vi "Clear IP.vi"(8 "error in (no error)":errorcluster, 11 "Engine Simulation IP in":refnum<class "Engine Simulation IP.lvclass">) -> (0 "error out":errorcluster)   [LabVIEW 2013, in "Engine Simulation IP.lvclass"]
uses:
  Engine Simulation IP.lvclass
  Engine Simulation IP.lvclass/Engine Simulation IP.ctl
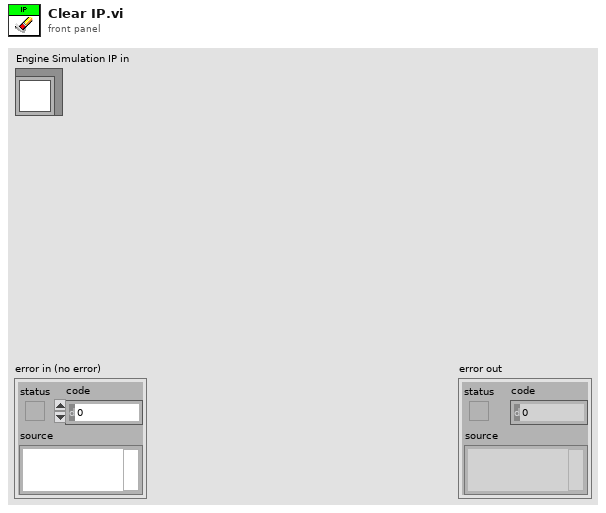
[diagram p1: front panel]
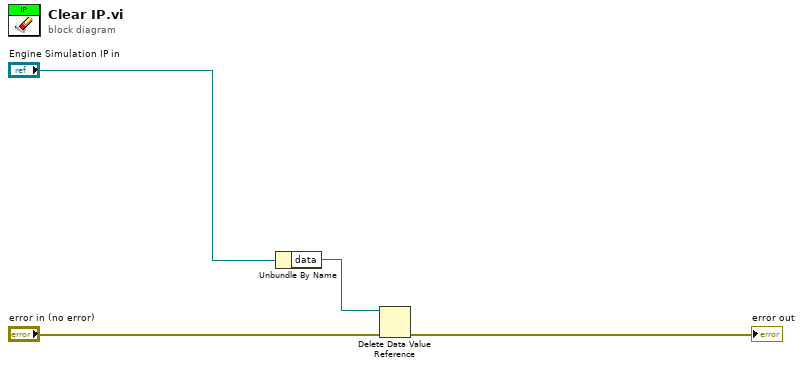
[diagram p0: block diagram]
diagram:
  n1 = Unbundle By Name("Engine Simulation IP in") -> ("data"=w1:refnum<data-value>)
  n2 = Delete Data Value Reference(data value reference=w1, error in="error in (no error)") -> (error out=→"error out":errorcluster)  [unwired: 1 out]
